vi "FPGA Main Default.vi"() -> ()   [LabVIEW 2014]
doc: "The myRIO v1.1 FPGA Shipping Personality. This personality contains support for:\n- 2 Analog Input Interrupt channel\n- 4 Digital Input Interrupt channel\n- 1 Timer\n- 1 Accelerometer\n- 1 Button\n- 4 LED\n- 10 Analog Input channels with 1 Sample\n- 6 Analog Output channels with 1 Sample\n- 40 Digital I/O channels with 1 Sample\n- 2 I2C channels\n- 4 Encoder channels\n- 6 PWM channels\n- 2 SPI channels"
uses:
  <vilib>/rvi/Emulation/niFpgaGetClockAttributes.vi
  <vilib>/rvi/Emulation/niFpgaSctlEmulationGetInTimedLoop.vi
  <vilib>/rvi/Emulation/niFpgaEmulationReportErrorSimple.vi
  <vilib>/rvi/eio/common/nirviEmuTemplateMethod_errors.vi
  <vilib>/rvi/Emulation/niFpgaCriticalErrorInLSC.vi
  <vilib>/eio/EIONode/EIONode.xnode
  Sub VIs/Maxim 1-Wire/Maxim 1-Wire.lvlib
panel:
  in  "DIO.A.DIO3":bool
  in  "DIO.A.DIO2":bool
  in  "DIO.A.DIO1":bool
  in  "DIO.A.DIO0":bool
  in  "DIO.A.DIO14":bool
  out "ROM Array":u64[](array[numeric]) format="%x"
  out "Temperature Array":u16[](array[numeric]) format="%x"
  in  "AO.A_0.VAL":u16
  in  "AO.A_1.VAL":u16
  in  "AO.B_0.VAL":u16
  in  "AO.B_1.VAL":u16
  out "AI.A_3.VAL":u16
  out "AI.A_2.VAL":u16
  out "AI.A_1.VAL":u16
  out "AI.A_0.VAL":u16
  in  "AO.C_0.VAL":u16
  in  "AO.C_1.VAL":u16
  out "AI.AudioIn_R.VAL":u16
  out "AI.AudioIn_L.VAL":u16
  in  "AO.AudioOut_R.VAL":u16
  in  "AO.AudioOut_L.VAL":u16
  # "System"
  # "Onboard Devices"
  # "Connector A"
  # "Connector B"
  # "Connector C"
  # "Audio Connector"
  # "Analog Input"
  # "Analog Output"
  # "1-Wire"
  # "Analog Input"
  # "Analog Output"
  # "Analog Input"
  # "Analog Output"
  # "Analog Input"
  # "Analog Output"
  # "Buttons & LEDs"
  # "Button Interrupt"
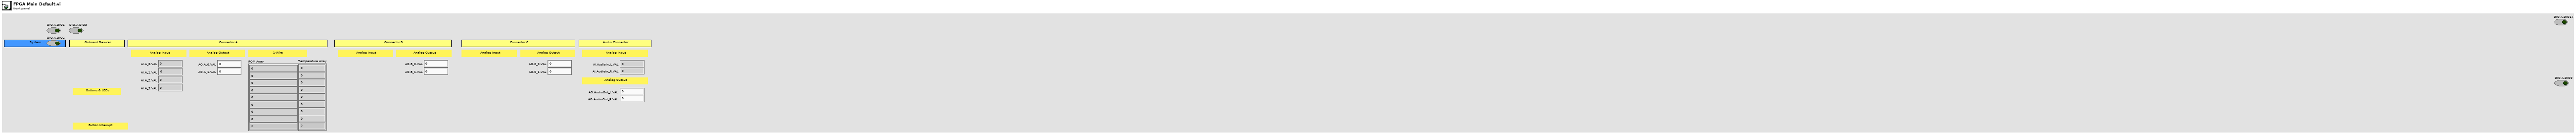
[diagram p1: front panel]
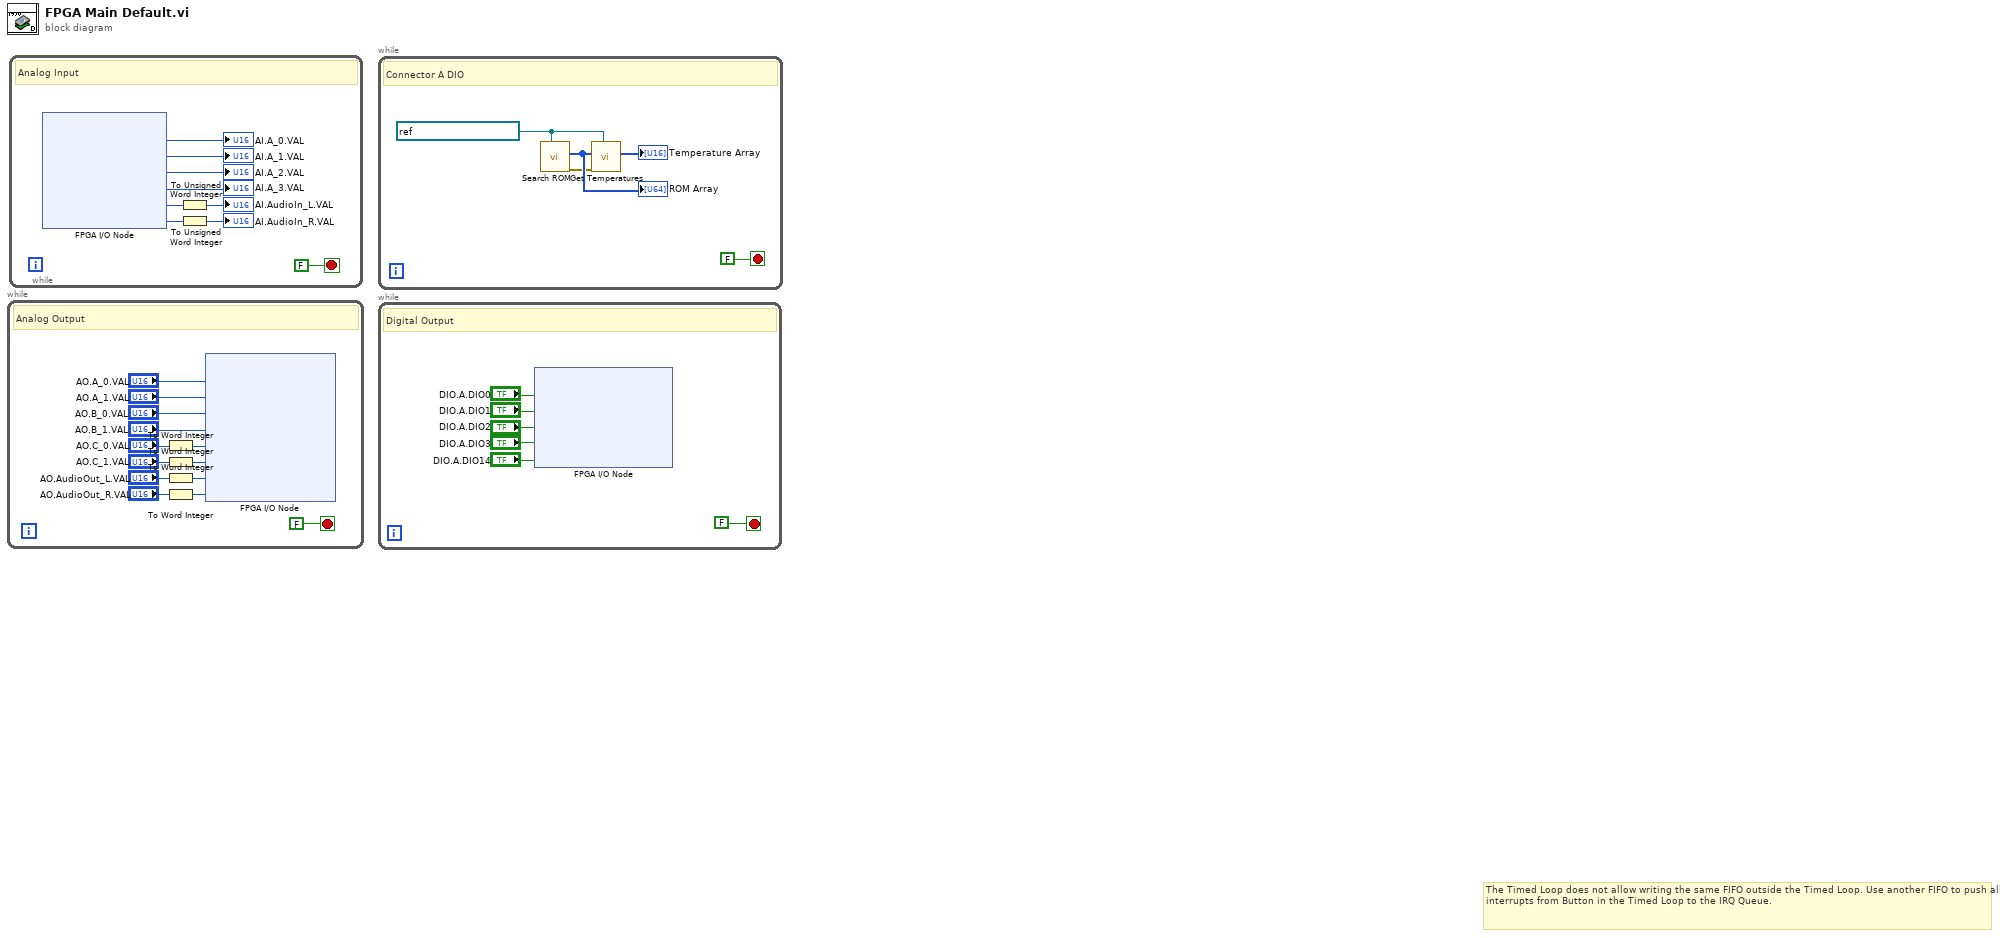
[diagram p0: block diagram]
diagram:
  # "The Timed Loop does not allow writing the same FIFO outside the Timed Loop. Use another FIFO to push all interrupts from Button in the Timed Loop to the IRQ Queue."
  n1 = while {
    stop <- FALSE stop-if-true
    # "Analog Output"
    n2 = To Word Integer(number="AO.C_0.VAL") -> (16bit integer=w4:i16)
    n3 = To Word Integer(number="AO.C_1.VAL") -> (16bit integer=w3:i16)
    n4 = To Word Integer(number="AO.AudioOut_L.VAL") -> (16bit integer=w2:i16)
    n5 = To Word Integer(number="AO.AudioOut_R.VAL") -> (16bit integer=w1:i16)
    n6 = xnode "FPGA I/O Node"("ConnectorA/AO0"="AO.A_0.VAL", "ConnectorA/AO1"="AO.A_1.VAL", "ConnectorB/AO0"="AO.B_0.VAL", "ConnectorB/AO1"="AO.B_1.VAL", "ConnectorC/AO0"=w4, "ConnectorC/AO1"=w3, "AudioOut/Left"=w2, "AudioOut/Right"=w1) -> ()  [unwired: 8 in, 8 out]
  }
  n7 = while {
    stop <- FALSE stop-if-true
    # "Analog Input"
    n8 = xnode "FPGA I/O Node"() -> ("ConnectorA/AI0"=→"AI.A_0.VAL":u16, "ConnectorA/AI1"=→"AI.A_1.VAL":u16, "ConnectorA/AI2"=→"AI.A_2.VAL":u16, "ConnectorA/AI3"=→"AI.A_3.VAL":u16, "AudioIn/Left"=w15:i16, "AudioIn/Right"=w14:i16)  [unwired: 6 in, 6 out]
    n9 = To Unsigned Word Integer(number=w15) -> (unsigned 16bit integer=→"AI.AudioIn_L.VAL":u16)
    n10 = To Unsigned Word Integer(number=w14) -> (unsigned 16bit integer=→"AI.AudioIn_R.VAL":u16)
  }
  n11 = while {
    stop <- FALSE stop-if-true
    w25 = refnum<k21> "ConnectorA/DIO15" ("1-Wire DIO Pin")
    # "Connector A DIO"
    n12 = call "Search ROM.vi"("1-Wire DIO Pin"=w25) -> ("Error Out"=w23:errorcluster, "ROM Array"=w24:u64[])  [unwired: 8 in, 1 out]
    "ROM Array" <- w24
    n13 = call "Get Temperatures.vi"("1-Wire DIO Pin"=w25, "error in (no error)"=w23, "ROM Array"=w24) -> ("Temperature Array"=→"Temperature Array":u16[])  [unwired: 7 in, 1 out]
  }
  n14 = while "Digital Outputs" {
    stop <- FALSE stop-if-true
    # "Digital Output"
    n15 = xnode "FPGA I/O Node"("ConnectorA/DIO0"="DIO.A.DIO0", "ConnectorA/DIO1"="DIO.A.DIO1", "ConnectorA/DIO2"="DIO.A.DIO2", "ConnectorA/DIO3"="DIO.A.DIO3", "ConnectorA/DIO14"="DIO.A.DIO14") -> ()  [unwired: 5 in, 5 out]
  }
